vi "Get_(X_Y_dX_dY)_from_Array-2.vi"(0 "(X,Y,dX,dY)":dbl[](array[numeric]), 1 "Index of Displacement":i32) -> (2 "X":dbl, 3 "Y":dbl, 4 "dX":dbl, 5 "dY":dbl)   [LabVIEW 2013]
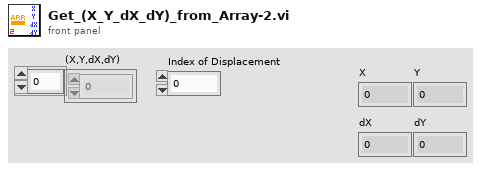
[diagram p1: front panel]
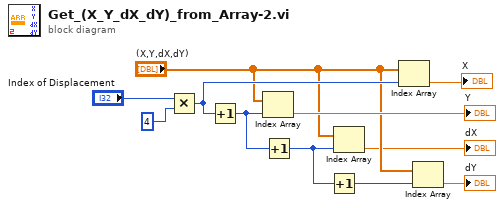
[diagram p0: block diagram]
diagram:
  n1 = Multiply(x="Index of Displacement", y=4 ("multiplier")) -> (x*y=w9:i32)
  n2 = Increment(x=w9) -> (x+1=w8:i32)
  n3 = Index Array(array="(X,Y,dX,dY)", index=w8) -> (element=→"Y":dbl)
  n4 = Increment(x=w8) -> (x+1=w6:i32)
  n5 = Increment(x=w6) -> (x+1=w4:i32)
  n6 = Index Array(array="(X,Y,dX,dY)", index=w6) -> (element=→"dX":dbl)
  n7 = Index Array(array="(X,Y,dX,dY)", index=w9) -> (element=→"X":dbl)
  n8 = Index Array(array="(X,Y,dX,dY)", index=w4) -> (element=→"dY":dbl)
